vi "DelayGenerator-StaticBaseline.vi"(3 "Time Stamp":timestamp, 9 "error in (no error)":errorcluster caption="error out") -> (0 "DelayTarget":T1, 6 "error out":errorcluster)   [LabVIEW 2009]
uses:
  Controls/DelayTarget.ctl
  <vilib>/Analysis/baseanly.llb/Real Dot Product.vi
  <vilib>/Analysis/NI_AALBase.lvlib
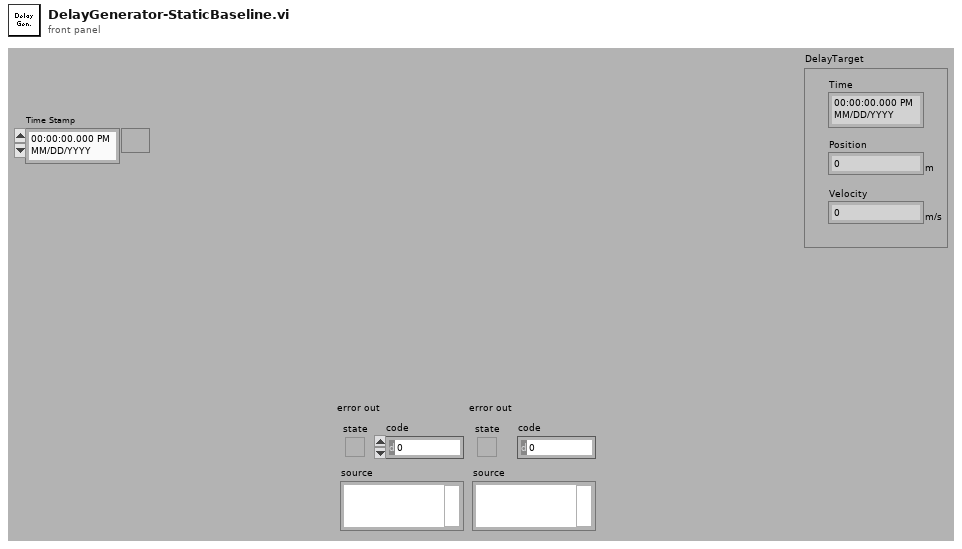
[diagram p1: front panel]
types:
  T1 = typedef "DelayTarget.ctl" = cluster{"Time":timestamp, "Position":dbl[unit], "Velocity":dbl[unit]}
  T2 = cluster{"latitude":dbl[unit], "longitude":dbl[unit], "height":dbl[unit], "temperature":dbl, "pressure":dbl}
  T3 = cluster{"East":dbl[unit], "North":dbl[unit], "Up":dbl[unit]}
  T4 = cluster{"catalog":string, "starname":string, "starnumber":i32, "ra":dbl[unit], "dec":dbl[unit], "promora":dbl[unit], "promodec":dbl[unit], "parallax":dbl[unit], "radialvelocity":dbl[unit]}
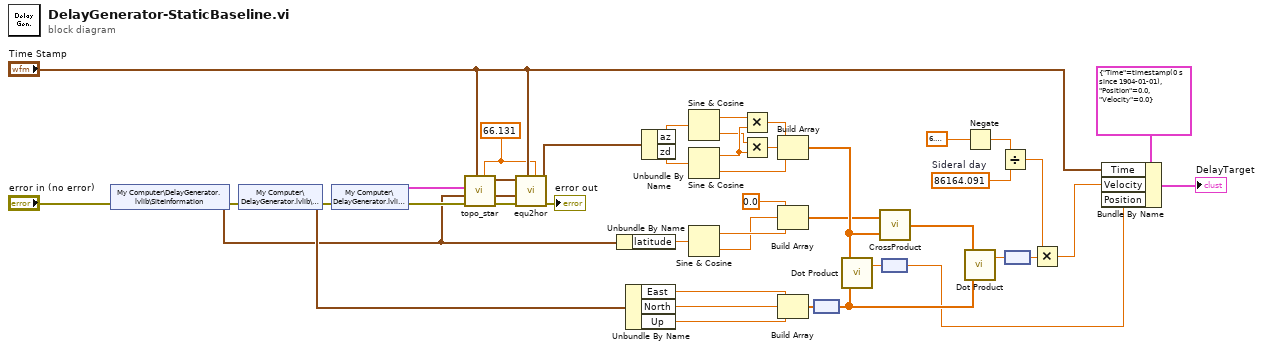
[diagram p0: block diagram]
diagram:
  w4 = dbl[unit] 66.131 ("dt")
  w18 = dbl[unit] 86164.091  # Sideral day
  n1 = shared-variable "My Computer\\DelayGenerator.lvlib\\SiteInformation"(error in="error in (no error)") -> (w2:T2, error out=w8:errorcluster)
  n2 = shared-variable "My Computer\\DelayGenerator.lvlib\\Baseline"(error in=w8) -> (w3:T3, error out=w7:errorcluster)
  n3 = shared-variable "My Computer\\DelayGenerator.lvlib\\Target"(error in=w7) -> (w1:T4, error out=w5:errorcluster)
  n4 = call "topo_star.vi"("deltat (TT-UT1)"=w4, "TimeStamp [UT1]"="Time Stamp", "error in (no error)"=w5, "on_surface"=w2, "cat_entry"=w1) -> ("error out"=w23:errorcluster, "ra/dec"=w24:cluster{"ra":dbl[unit], "dec":dbl[unit]})  [unwired: 3 in]
  n5 = call "equ2hor.vi"("deltat [TT-UT1]"=w4, "TimeStamp [UT1]"="Time Stamp", "error in (no error)"=w23, "on_surface"=w2, "ra/dec"=w24) -> ("error out"=→"error out":errorcluster, "az/zd"=w22:cluster{"az":dbl[unit], "zd":dbl[unit]})  [unwired: 2 in, 1 out]
  n6 = Unbundle By Name(w2) -> ("latitude"=w39:dbl[unit])
  n7 = Unbundle By Name(w3) -> ("East"=w28:dbl[unit], "North"=w27:dbl[unit], "Up"=w29:dbl[unit])
  n8 = Unbundle By Name(w22) -> ("az"=w38:dbl[unit], "zd"=w31:dbl[unit])
  n9 = Sine & Cosine(0:w38) -> (1:w33:dbl, 2:w32:dbl)
  n10 = Sine & Cosine(0:w31) -> (1:w34:dbl, 2:w37:dbl)
  n11 = Sine & Cosine(0:w39) -> (1:w21:dbl, 2:w20:dbl)
  n12 = Multiply(x=w33, y=w34) -> (x*y=w35:dbl)
  n13 = Multiply(x=w32, y=w34) -> (x*y=w36:dbl)
  n14 = Build Array(w35, w36, w37) -> (w19:dbl[])
  n15 = Build Array(0.0 ("élément"), w20, w21) -> (w16:dbl[])
  n16 = Build Array(w28, w27, w29) -> (w26:dbl[unit][])
  n17 = node(w26) -> (w43:dbl[])
  n18 = call-poly <vilib>:"Dot Product.vi"("Y Vector"=w43, "X Vector"=w19) -> ("X * Y"=w30:dbl)  [unwired: 1 out]
  n19 = call "CrossProduct.vi"("V2"=w19, "V1"=w16) -> ("V1^V2"=w42:dbl[])
  n20 = node(w30) -> (w11:dbl[unit])
  n21 = Negate(x=6.283185307179586) -> (-x=w14:dbl)
  n22 = call-poly <vilib>:"Dot Product.vi"("Y Vector"=w43, "X Vector"=w42) -> ("X * Y"=w41:dbl)  [unwired: 1 out]
  n23 = Divide(x=w14, y=w18) -> (x/y=w17:dbl[unit])
  n24 = node(w41) -> (w44:dbl[unit])
  n25 = Multiply(x=w17, y=w44) -> (x*y=w10:dbl[unit])
  n26 = Bundle By Name(cluster=T1 {"Time"=timestamp(0 s since 1904-01-01), "Position"=0.0, "Velocity"=0.0} ("DelayTarget"), "Time"="Time Stamp", "Velocity"=w10, "Position"=w11) -> (→"DelayTarget":T1)
